vi "Generate AIM API Errors.vi"() -> ()   [LabVIEW 2020]
uses:
  <instrlib>/AIM GmbH/_ARINC-429/VIs/Library/Api429Lib Error Desc Get.vi
  <instrlib>/AIM GmbH/_ARINC-429/subvi/Get Error Number Offset.vi
  <instrlib>/AIM GmbH/_ARINC-429/subvi/Get Library Path.vi
  <vilib>/Utility/error.llb/Error Cluster From Error Code.vi
  <instrlib>/AIM GmbH/_ARINC-429/AIM429LV.lvlib
panel:
  out "error file text":string
  in  "header":string="<?xml version=\"1.0\" encoding=\"ISO-8859-1\"?>\n<nidocument>\n<nicomment>\nErrors generated from AIM429LV.lilb:Error Converter (ErrCode or Status).vi.\nhttps://github.com/ni/niveristand-aim-arinc429-custom-device/\n</nicomment>\n"
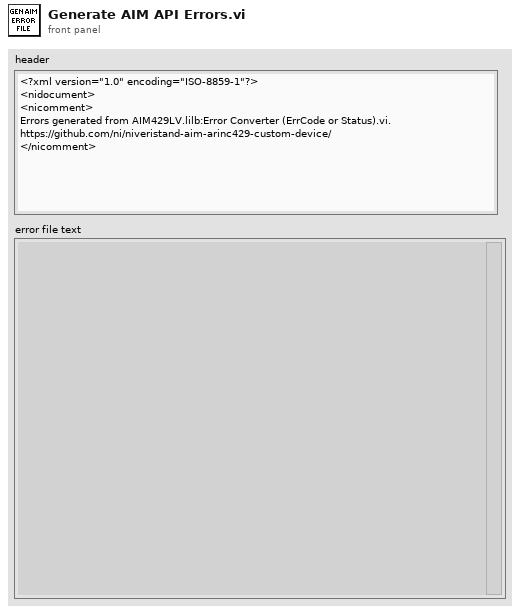
[diagram p1: front panel]
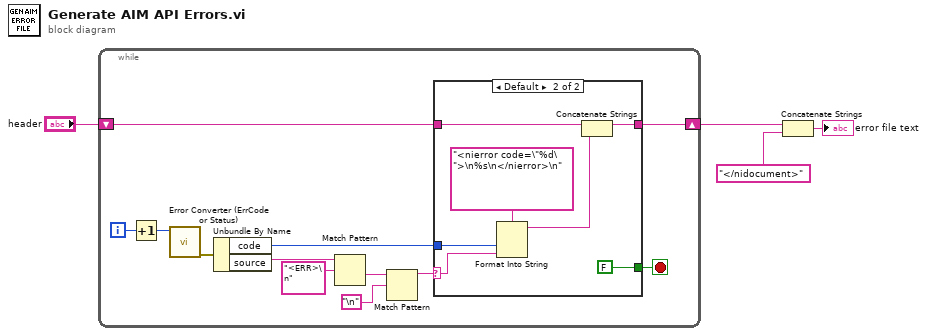
[diagram p0: block diagram]
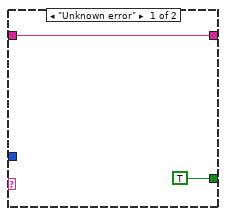
[diagram p2: hidden frame]
diagram:
  n1 = while {
    shift-right: [w13] -> w3
    shift-left: "header" -> [w14]
    i -> [w7]
    stop <- w5 stop-if-true
    n2 = Increment(x=w7) -> (x+1=w8:i32)
    n3 = call <instrlib>:"Error Converter (ErrCode or Status).vi"("error code"=w8) -> ("error out"=w16:errorcluster)  [unwired: 10 in]
    n4 = Unbundle By Name(w16) -> ("code"=w15:i32, "source"=w12:string)
    n5 = Match Pattern(string=w12, regular expression="<ERR>\n") -> (after substring=w9:string)  [unwired: 1 in, 3 out]
    n6 = Match Pattern(string=w9, regular expression="\n") -> (before substring=w6:string)  [unwired: 1 in, 3 out]
    n7 = case shown="Default" w6 {
      selector: w6 -> [_ w19]
      tunnel: w15 -> [_ w24]
      tunnel: w14 -> [w18 w23]
      tunnel: [w18 w21] -> w13
      tunnel: [TRUE FALSE] -> w5
      frame "Unknown error" {
      }
      frame Default {
        n8 = Format Into String(format string="<nierror code=\"%d\">\n%s\n</nierror>\n", w24, w19) -> (resulting string=w22:string)  [unwired: 2 in, 1 out]
        n9 = Concatenate Strings(w23, w22) -> (w21:string)
      }
    }
  }
  n10 = Concatenate Strings(w3, "</nidocument>" ("string")) -> (→"error file text":string)
